vi "Generate Log Record (Internal).vi"(6 "populate call chain? (F)":bool, 7 "call chain elements to ignore (0)":i32, 9 "data (null)":variant, 10 "message (\"\")":string, 11 "level (Internal)":T2=enum."Internal") -> (3 "log record":T1 {"timestamp" format="%<%x %.3X>T"})   [LabVIEW 2018, in "GLog.lvlib" / "Logger.lvclass"]
uses:
  Logger.lvclass
  Internal Log Levels.ctl
  Log Record.ctl
  GLog.lvlib
panel:
  # "Connector Pane"
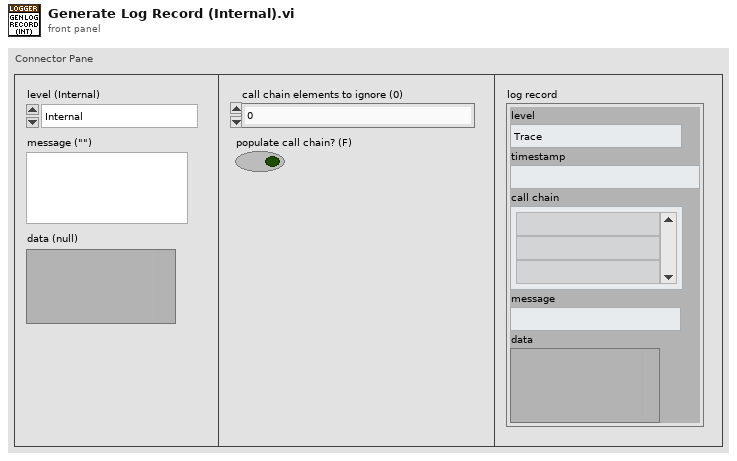
[diagram p1: front panel]
types:
  T1 = typedef "GLog.lvlib/Log Record.ctl" = cluster{"level":T2, "timestamp":timestamp, "call chain":string[], "message":string, "data":variant}
  T2 = typedef "GLog.lvlib/Internal Log Levels.ctl" = enum16{"Trace", "Debug", "Info", "Warning", "Error", "Critical", "Internal"}
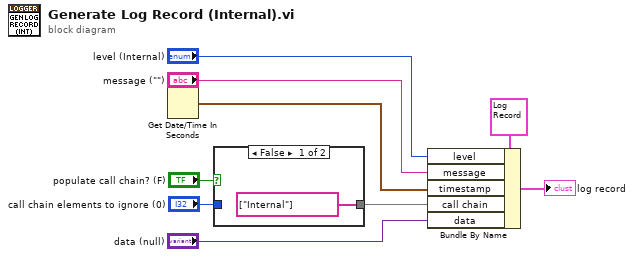
[diagram p0: block diagram]
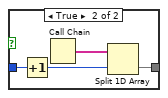
[diagram p2: hidden frame]
diagram:
  n1 = Get Date/Time In Seconds() -> (seconds since 1Jan1904=w9:timestamp)
  n2 = case shown="False" "populate call chain? (F)" {
    tunnel: [string[] ["Internal"] w13] -> w3
    tunnel: "call chain elements to ignore (0)" -> [_ w11]
    frame False {
    }
    frame True {
      n3 = Increment(x=w11) -> (x+1=w12:i32)
      n4 = Call Chain() -> (call chain=w14:string[])
      n5 = Split 1D Array(array=w14, index=w12) -> (second subarray=w13:string[])  [unwired: 1 out]
    }
  }
  n6 = Bundle By Name(cluster=T1 {"level"=enum."Trace", "timestamp"=timestamp(0 s since 1904-01-01), "call chain"=[], "message"="", "data"=variant} ("output cluster 2"), "level"="level (Internal)", "message"="message (\"\")", "timestamp"=w9, "call chain"=w3, "data"="data (null)") -> (→"log record":T1)
